vi "Build Toolkit VIs.vi"(5 "Project File":path, 7 "Target Version":string="15.0", 8 "Error In":errorcluster) -> (0 "Error Out":errorcluster)   [LabVIEW 2017]
uses:
  <vilib>/AppBuilder/AB_API_Simple/Build (path).vi
  <vilib>/AppBuilder/AB_API_Simple/NI_App_Builder_API.lvlib
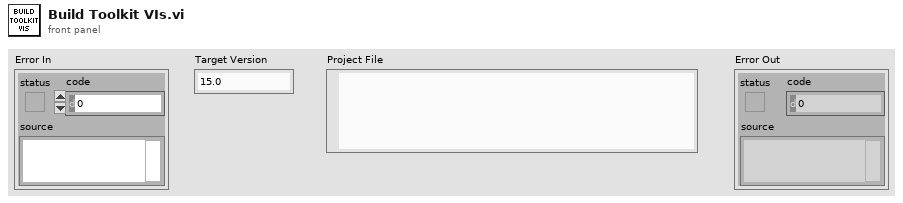
[diagram p1: front panel]
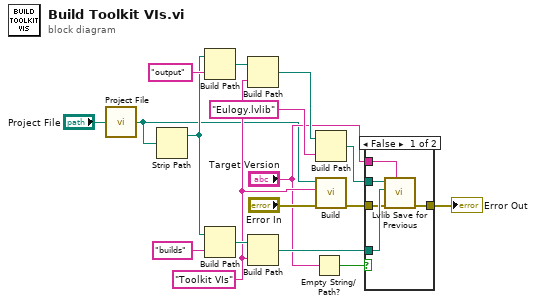
[diagram p0: block diagram]
diagram:
  w9 = "Toolkit VIs" ("name or relative path")
  n1 = call "Project File.vi"("Project File In"="Project File") -> ("Project File Out"=w1:path)
  n2 = Strip Path(path=w1) -> (stripped path=w5:path)  [unwired: 1 out]
  n3 = Build Path(base path=w5, name or relative path="output") -> (appended path=w16:path)
  n4 = Build Path(base path=w5, name or relative path="builds") -> (appended path=w11:path)
  n5 = Build Path(base path=w16, name or relative path=w9) -> (appended path=w15:path)
  n6 = Build Path(base path=w11, name or relative path=w9) -> (appended path=w10:path)
  n7 = Empty String/Path?(string/path="Target Version") -> (empty?=w3:bool)
  n8 = Build Path(base path=w15, name or relative path="Eulogy.lvlib") -> (appended path=w13:path)
  n9 = call-poly <vilib>:"Build.vi"("error in (no error)"="Error In", "Name of build specification (if empty: build all)"=w9, "Path to project"=w1) -> ("error out"=w8:errorcluster)  [unwired: 7 in, 1 out]
  n10 = case shown="False" w3 {
    tunnel: w13 -> [w22 _]
    tunnel: w10 -> [w21 _]
    tunnel: w8 -> [w20 w23]
    tunnel: [w19 w23] -> w6
    tunnel: "Target Version" -> [w18 _]
    frame False {
      n11 = call "Lvlib Save for Previous.vi"("Target Version"=w18, "Error In"=w20, "Destination Folder"=w21, "Original lvlib"=w22) -> ("Error Out"=w19:errorcluster)  [unwired: 7 in]
    }
    frame True {
    }
  }
  "Error Out" <- w6
